vi "FilterTest Setup.vi"(8 "error in (no error)":errorcluster, 10 "Number of Test Filters":i32=2) -> (0 "error out":errorcluster, 3 "Main Display out":refnum<class "Main Display.lvclass">)   [LabVIEW 2016, in "Assert API Components.lvlib" / "Assert Display.lvlib" / "Main Display.lvlib" / "Main Display.lvclass"]
uses:
  Main Display.lvclass
  Assert API Components/Filter Configurations/Base Filter.lvclass
  Assert API Components/Filter Configurations/Base Filter.lvclass/Base Filter.ctl
  Main Display.lvclass/Main Display.ctl
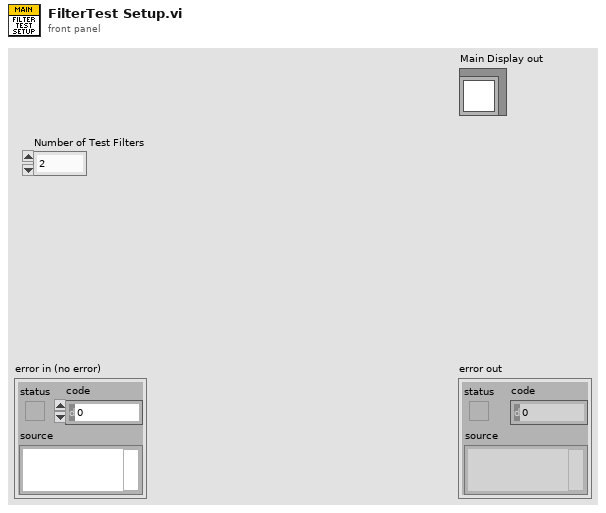
[diagram p1: front panel]
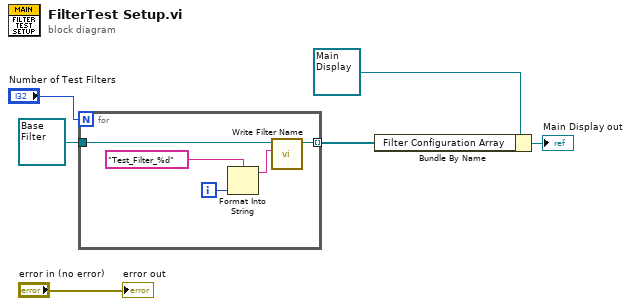
[diagram p0: block diagram]
diagram:
  n1 = for {
    N: "Number of Test Filters" -> [_]
    tunnel: refnum<class "Base Filter.lvclass"> refnum ("Assert API Components.lvlib:Base Filter.lvclass") -> [w11]
    tunnel: [w7] -> w1 mode=indexing
    i -> [w10]
    n2 = Format Into String(format string="Test_Filter_%d", w10) -> (resulting string=w8:string)  [unwired: 2 in, 1 out]
    n3 = call "Write Filter Name.vi"("Filter Name"=w8, "Base Filter in"=w11) -> ("Base Filter out"=w7:refnum<class "Base Filter.lvclass">)  [unwired: 9 in]
  }
  n4 = Bundle By Name(cluster=refnum<class "Main Display.lvclass"> refnum ("Main Display in"), "Filter Configuration Array"=w1) -> (→"Main Display out":refnum<class "Main Display.lvclass">)
  "error out" <- "error in (no error)"
